vi "Aimed Navigation.vi"() -> ()   [LabVIEW 2020]
uses:
  command.ctl
  <vilib>/regexp/Match Regular Expression.xnode
panel:
  out "Answer":i32
  in  "Input":string="forward 1\ndown 6\ndown 6\nforward 2\nforward 2\ndown 2\ndown 1\ndown 5\ndown 7\ndown 3\nforward 1\nforward 6\nup 2\nforward 2\nforward 7\nforward 4\ndown 2\nforward 6\nforward 6\ndown 3\nup 7\ndown 6\nforward 2\nup 5\ndown 7\nforward 8\ndown 8\nforward 8\ndown 5\ndown 5\ndown 8\nforward 9\ndown 7\nforward 9\nforward 9\nforward 8\ndown 6\ndown 9\ndown 1\nforward 8\ndown 6\ndown 7\nup 3\nforward 5\ndown 1\ndown 7\nup 8\nforward 6\ndown 2\ndown 9\ndown 9\nforward 1\ndown 2\ndown 9\nforward 1\nforward 3\ndown 6\nup 7\ndown 7\nforward 3\ndown 4\ndown 3\nup 7\nup 7\nforward 2\ndown 7\nforward 2\ndown 3\nup 7\ndown 7\nforward 6\ndown 2\ndown 7\nforward 5\ndown 9\ndown 2\nup 7\ndown 1\nforward 5\ndown 5\nforward 9\ndown 6\ndown 3\ndown 7\ndown 8\ndown 3\nup 4\ndown 6\nforward 6\nup 7\nup 2\nforward 3\nup 1\ndown 5\nforward 9\nup 3\nforward 8\nup 4\ndown 7\ndown 8\ndown 3\ndown 7\nforward 5\nup 6\ndown 4\ndown 8\ndown 8\nforward 7\ndown 5\nforward 3\nforward 1\ndown 1\nforward 1\nup 1\nforward 4\nforward 9\nup 8\ndown 7\ndown 9\ndown 1\ndown 2\ndown 1\ndown 4\nforward 4\nforward 8\nforward 6\nforward 1\nforward 6\nforward 9\ndown 1\nup 9\ndown 9\nforward 2\ndown 6\ndown 8\ndown 6\nup 7\nforward 2\nup 2\nforward 5\ndown 2\nup 2\nup 9\nforward 7\ndown 6\nforward 3\ndown 5\nup 4\ndown 1\ndown 5\ndown 6\nup 7\ndown 3\ndown 9\nup 8\ndown 2\nup 8\ndown 1\ndown 2\ndown 4\nforward 6\nup 7\nup 3\nforward 8\ndown 9\ndown 8\nforward 3\nup 5\nforward 1\ndown 5\nup 2\ndown 5\nup 4\ndown 6\nforward 9\ndown 1\ndown 1\nforward 1\ndown 2\nforward 9\nup 5\ndown 7\nforward 7\ndown 9\ndown 5\ndown 3\nforward 4\ndown 2\nforward 7\nforward 3\nup 4\ndown 9\nforward 9\nforward 3\nforward 1\nforward 6\ndown 1\ndown 5\ndown 3\nforward 9\ndown 2\nforward 9\nup 7\nforward 7\nforward 7\nforward 8\nforward 6\nforward 5\ndown 7\nup 4\nforward 7\nup 2\nforward 6\ndown 2\ndown 9\ndown 3\nforward 5\ndown 3\ndown 9\nforward 2\nup 4\nforward 7\nforward 3\nforward 8\ndown 4\nforward 4\ndown 3\nup 7\nup 1\nup 4\ndown 3\ndown 5\ndown 3\ndown 7\ndown 3\ndown 7\ndown 5\ndown 1\nforward 5\nforward 6\ndown 1\nforward 9\ndown 4\nup 1\nforward 5\nup 6\ndown 4\nup 7\ndown 4\ndown 9\nforward 7\nup 8\nforward 3\nforward 5\ndown 9\ndown 1\ndown 7\nforward 9\ndown 9\ndown 5\nforward 6\nforward 4\nforward 3\ndown 1\ndown 2\nup 4\nup 7\ndown 8\nforward 4\nforward 1\nforward 8\ndown 8\ndown 8\nforward 1\nforward 5\nup 8\nforward 2\ndown 6\nforward 6\ndown 6\nforward 7\ndown 9\ndown 4\nup 4\nup 5\ndown 7\nforward 4\ndown 7\ndown 5\nforward 7\ndown 3\ndown 2\nforward 5\nforward 1\ndown 5\ndown 4\ndown 8\nup 8\nforward 3\ndown 7\ndown 8\ndown 5\nforward 1\ndown 6\nforward 8\nforward 2\nforward 3\ndown 4\nup 3\ndown 4\nforward 3\nforward 9\nup 5\nup 9\ndown 3\nup 4\nforward 4\ndown 9\nforward 8\ndown 2\ndown 2\nforward 9\ndown 5\ndown 2\nup 1\nforward 6\nforward 4\nup 5\nup 3\nup 8\ndown 7\nforward 5\nup 7\nforward 9\ndown 6\ndown 7\nforward 4\ndown 9\nup 2\nforward 8\ndown 1\nforward 6\nforward 1\nforward 4\ndown 9\ndown 6\nup 1\nforward 1\ndown 5\nup 1\nforward 3\ndown 1\ndown 4\nforward 3\ndown 4\nup 9\ndown 6\nup 6\nforward 1\nforward 8\nup 1\ndown 7\nup 8\nup 3\nup 7\ndown 9\nforward 8\ndown 3\nup 2\nforward 3\nup 4\nup 3\ndown 5\nforward 3\nforward 2\ndown 3\nforward 5\nup 4\ndown 9\ndown 8\ndown 3\ndown 5\ndown 7\nforward 2\nforward 8\nup 9\nforward 9\ndown 4\ndown 8\nforward 5\ndown 2\nup 4\ndown 7\nforward 6\nup 9\nforward 6\ndown 9\ndown 5\nforward 9\ndown 5\ndown 3\nup 6\nup 6\ndown 7\nup 1\nforward 7\nforward 4\ndown 5\nforward 8\ndown 5\ndown 8\nforward 4\nforward 8\nforward 1\ndown 7\nforward 4\ndown 6\ndown 4\nup 8\ndown 4\nup 5\nup 7\nup 2\ndown 5\ndown 9\nforward 6\ndown 7\ndown 9\ndown 3\nup 4\ndown 8\nforward 3\nforward 5\nforward 8\ndown 9\nforward 9\ndown 1\nup 1\ndown 9\nforward 3\nup 9\nforward 5\nforward 2\ndown 1\ndown 5\ndown 6\nforward 5\nforward 4\nup 5\nforward 5\nup 4\nup 9\nup 4\nforward 8\ndown 7\ndown 6\ndown 9\ndown 3\ndown 2\ndown 6\nup 6\nforward 6\nup 3\ndown 3\nforward 3\ndown 2\ndown 9\ndown 3\nforward 1\nforward 8\ndown 2\ndown 9\ndown 6\nup 3\ndown 6\nforward 1\nforward 1\nforward 2\ndown 9\ndown 8\nforward 9\ndown 2\nup 3\nforward 2\nup 5\nup 8\ndown 4\nup 3\nforward 3\nforward 5\nforward 1\ndown 5\nup 4\nforward 4\ndown 7\nforward 8\nup 7\nforward 5\ndown 2\nforward 4\nforward 6\ndown 7\ndown 9\nforward 2\nforward 2\ndown 4\ndown 5\nup 5\nforward 5\nforward 2\ndown 8\nforward 6\ndown 1\ndown 6\nforward 1\ndown 8\nup 6\ndown 8\nforward 4\ndown 4\ndown 4\nforward 3\nup 8\ndown 1\nforward 7\ndown 5\nforward 1\ndown 9\ndown 9\ndown 5\nforward 1\ndown 4\nup 6\nforward 4\nforward 5\nforward 1\ndown 4\ndown 2\ndown 5\nforward 6\nforward 1\nforward 6\ndown 2\ndown 6\nforward 3\ndown 9\nup 6\nforward 2\nup 7\nforward 8\ndown 7\nup 1\nforward 1\ndown 8\nforward 8\ndown 9\nforward 4\ndown 4\ndown 5\ndown 8\nup 3\nforward 1\nforward 9\ndown 9\nup 2\ndown 1\ndown 8\ndown 6\nforward 3\ndown 8\ndown 3\nforward 5\nforward 2\nforward 5\nforward 5\nforward 2\nforward 4\ndown 9\ndown 3\nforward 7\nforward 3\nup 3\nup 1\nforward 2\ndown 5\nforward 3\nup 3\nforward 2\nforward 9\nforward 5\ndown 3\nforward 9\nup 2\nforward 7\nup 3\ndown 8\nforward 7\nup 5\nforward 3\nforward 4\nup 5\ndown 6\nup 2\nforward 8\nup 3\ndown 5\ndown 4\nforward 9\nup 2\ndown 5\nforward 4\nup 7\ndown 9\nup 8\ndown 4\nup 5\nforward 4\ndown 8\nforward 3\ndown 5\ndown 5\ndown 8\nup 9\nforward 3\nforward 9\ndown 2\nforward 4\ndown 1\nup 3\ndown 9\nup 6\ndown 1\ndown 1\ndown 5\ndown 1\ndown 7\nforward 4\ndown 4\ndown 9\nup 1\nup 7\nup 2\ndown 8\nup 5\ndown 6\nforward 6\nforward 6\ndown 4\nforward 9\nforward 4\nforward 9\nforward 4\nup 5\nforward 9\nup 7\nup 1\nforward 5\nforward 9\ndown 7\nforward 7\nforward 6\ndown 5\nforward 9\nup 9\ndown 4\ndown 9\ndown 2\nforward 3\ndown 3\ndown 3\nforward 9\ndown 8\ndown 4\ndown 8\ndown 6\ndown 6\ndown 9\nup 5\ndown 3\ndown 4\nup 6\nup 2\nforward 1\nup 9\nup 9\nforward 9\nforward 7\ndown 3\nforward 2\nup 5\ndown 2\nforward 2\nforward 8\ndown 8\nforward 4\nforward 2\nup 3\nup 8\ndown 5\nforward 5\nforward 8\ndown 1\ndown 8\nforward 3\nforward 9\ndown 7\nforward 5\nforward 8\nforward 1\nup 6\nforward 9\nup 5\nforward 8\nforward 3\ndown 2\nup 9\nup 7\nforward 5\ndown 8\ndown 3\nforward 8\ndown 3\ndown 9\ndown 9\nforward 7\ndown 9\nforward 5\nforward 1\nforward 5\ndown 2\ndown 7\nforward 4\ndown 4\nup 8\ndown 2\nup 1\ndown 1\nup 5\nup 6\ndown 5\nup 9\nup 6\ndown 6\ndown 4\ndown 3\nforward 9\nforward 2\nforward 2\nup 6\nforward 9\ndown 3\nforward 4\nforward 6\nforward 8\nforward 2\nforward 8\nforward 4\ndown 1\nforward 3\nup 1\nup 9\nforward 9\nup 6\nup 5\nforward 2\ndown 6\nup 8\nup 9\nforward 3\nforward 9\ndown 7\ndown 6\nforward 2\ndown 7\nforward 4\ndown 5\ndown 2\ndown 6\ndown 2\ndown 5\ndown 3\nforward 3\ndown 7\ndown 6\ndown 5\nup 2\nforward 4\nup 9\nforward 2\nforward 4\ndown 5\nup 9\nup 2\nforward 9\nforward 6\ndown 6\ndown 3\ndown 5\ndown 1\nup 4\nup 1\ndown 4\ndown 1\nforward 5\nforward 3\ndown 7\ndown 9\nforward 2\ndown 3\nup 7\ndown 2\ndown 6\nforward 3\nforward 3\ndown 3\nup 1\nforward 6\nforward 3\ndown 6\ndown 2\nup 4\nup 3\ndown 5\ndown 9\ndown 3\nforward 7\nforward 2\nforward 9\ndown 6\nforward 4\nup 9\nforward 1\ndown 4\ndown 6\ndown 2\nforward 3\ndown 2\nup 8\nforward 1\nforward 9\ndown 9\nup 7\nforward 6\nup 8\ndown 9\ndown 4\nforward 8\ndown 6\ndown 1\ndown 9\ndown 1\nup 7\nforward 9\nup 3\nforward 7\nup 7\ndown 2\nforward 1\ndown 4\ndown 7\nforward 7\nforward 9\ndown 6\ndown 5\ndown 8\ndown 9\nup 3\ndown 7\nup 3\ndown 1\nforward 1\nforward 6\nforward 2\ndown 6\nforward 9\nforward 1\nup 2\nforward 1\nforward 3\nforward 4\nforward 7\nforward 4\ndown 3\nup 8\nforward 9\ndown 7\nforward 6\nforward 3\ndown 6\nforward 4\nup 1\nforward 3\ndown 3\nforward 9\nforward 2\nforward 1\nforward 4\nup 6\nforward 3\ndown 6\ndown 8\nup 4\nforward 8\nforward 4\ndown 8\nup 4\nup 3\nforward 9\nforward 3\ndown 5\nforward 7\nforward 1\nup 8\nup 4\ndown 1\ndown 3\ndown 9\ndown 7\nup 5\nforward 6\ndown 1\nforward 3\ndown 2\ndown 2\ndown 6\nforward 2\ndown 5\nforward 2\nforward 1\nup 9\ndown 1\nforward 3\ndown 3\nforward 6\ndown 1\nforward 5\nforward 7\ndown 6\nforward 7\ndown 4\nup 7\nforward 1\ndown 7\ndown 8\ndown 9\ndown 6\ndown 1\nforward 6\ndown 7\nforward 2\ndown 2\nup 1\nup 2\ndown 3\ndown 4\nup 2\nforward 3\ndown 5\ndown 4\ndown 9\ndown 6\ndown 9\ndown 7\ndown 2\nforward 7\nforward 3\nup 3\ndown 1\ndown 5\ndown 1\ndown 3\ndown 3\nforward 9\ndown 1\ndown 7\nup 4\ndown 1\ndown 6\nup 9\ndown 9\nforward 6\ndown 9\nforward 3\nforward 8\nup 1\nforward 3\ndown 8\nforward 2\ndown 6\ndown 1\nup 7\ndown 1\nforward 3\ndown 2\nforward 1\nup 8\nforward 8\nforward 7\ndown 9\nforward 3"
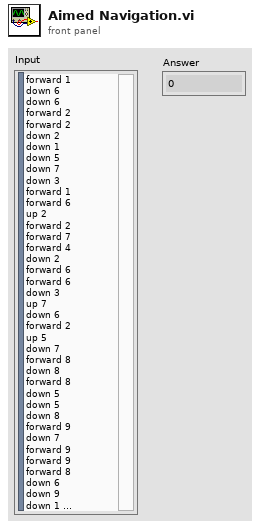
[diagram p1: front panel]
types:
  T1 = typedef "command.ctl" = enum16{"forward", "down", "up"}
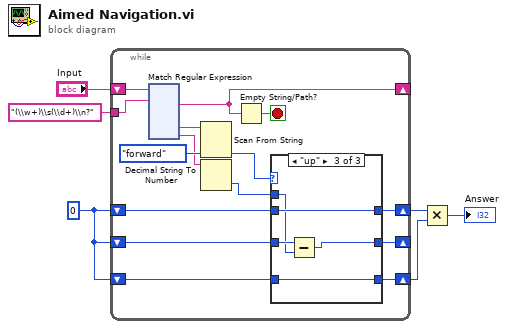
[diagram p0: block diagram]
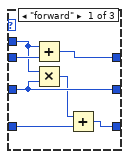
[diagram p2: hidden frame]
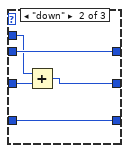
[diagram p3: hidden frame]
diagram:
  w2 = 0
  n1 = while {
    shift-right: [w19] -> _
    shift-left: "Input" -> [w21]
    tunnel: "(\\w+)\\s(\\d+)\\n?" -> [w20]
    shift-right: [w9] -> w4
    shift-left: w2 -> [w12]
    shift-right: [w10] -> _
    shift-left: w2 -> [w11]
    shift-right: [w7] -> w1
    shift-left: w2 -> [w8]
    stop <- w18 stop-if-true
    n2 = xnode "Match Regular Expression"("input string"=w21, "regular expression"=w20) -> ("after match"=w19:string, "submatch 1"=w17:string, "submatch 2"=w15:string)  [unwired: 4 in, 4 out]
    n3 = Scan From String(input string=w17, default 1=command."forward" ("command")) -> (output 1=w14:T1)  [unwired: 3 in, 3 out]
    n4 = Decimal String To Number(string=w15) -> (number=w13:i32)  [unwired: 2 in, 1 out]
    n5 = Empty String/Path?(string/path=w19) -> (empty?=w18:bool)
    n6 = case shown="\"up\"" w14 {
      tunnel: w13 -> [w25 w31 w36]
      tunnel: w12 -> [w28 w33 w38]
      tunnel: w11 -> [w26 w32 w37]
      tunnel: [w26 w30 w35] -> w10
      tunnel: [w27 w33 w38] -> w9
      tunnel: w8 -> [w24 w29 w34]
      tunnel: [w22 w29 w34] -> w7
      frame "forward" {
        n7 = Add(x=w25, y=w28) -> (x+y=w27:i32)
        n8 = Multiply(x=w25, y=w26) -> (x*y=w23:i32)
        n9 = Add(x=w23, y=w24) -> (x+y=w22:i32)
      }
      frame "down" {
        n10 = Add(x=w31, y=w32) -> (x+y=w30:i32)
      }
      frame "up" {
        n11 = Subtract(x=w37, y=w36) -> (x-y=w35:i32)
      }
    }
  }
  n12 = Multiply(x=w4, y=w1) -> (x*y=→"Answer":i32)
